vi "GetCtlRef_Base.vi"(8 "error in (no error)":errorcluster, 10 "Control Label":string, 11 "CtlLookup In":T1) -> (0 "error out":errorcluster, 2 "CtlRef Out":refnum<vi>, 3 "CtlLookup Out":T1)   [LabVIEW 2018, in "CtlReferences.lvlib" / "CtlReferences.lvclass"]
doc: "This is the base of the polymorphic VI \"GetControlRef\" \n\nThis is a General Helper VI.\n\nThis will search the incoming \"Ref Cluster\" for the Control Label string. If it finds it, it will output the reference If it does not, it will create an error -8000 with the control name"
uses:
  CtlReferences.lvclass
  TypeDefs/CtlLookup.ctl
  CtlReferences.lvclass/CtlReferences.ctl
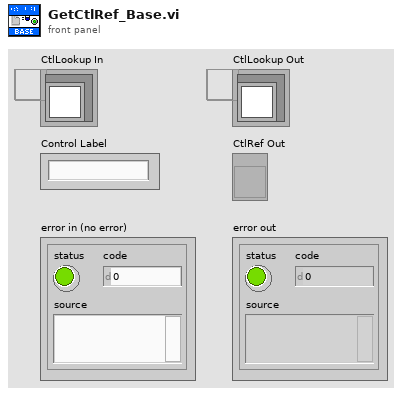
[diagram p1: front panel]
types:
  T1 = typedef "CtlReferences.lvlib/CtlReferences.lvclass/CtlLookup.ctl" = refnum<data-value>
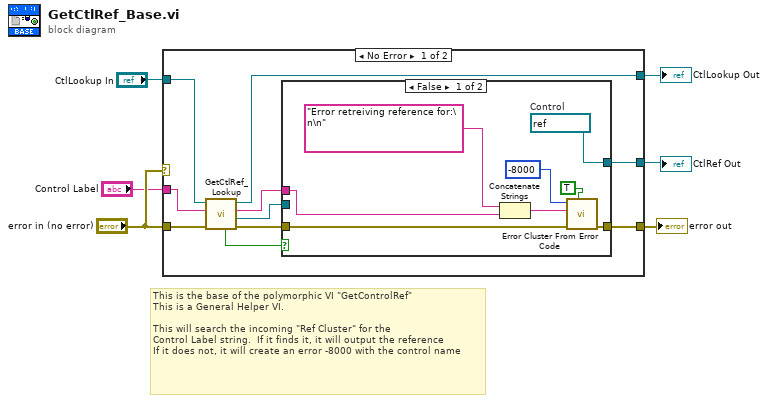
[diagram p0: block diagram]
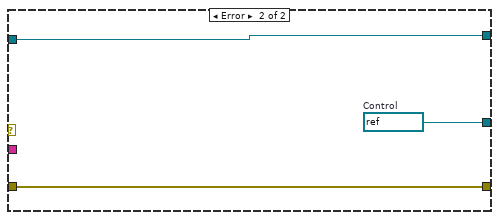
[diagram p3: hidden frame]
diagram:
  # "This is the base of the polymorphic VI \"GetControlRef\"\nThis is a General Helper VI.\n\nThis will search the incoming \"Ref Cluster\" for the \nControl Label string.  If it finds it, it will output the reference\nIf it does not, it will create an error -8000 with the control name"
  n1 = case shown="No Error" "error in (no error)" {
    tunnel: [w16 w29] -> w6
    tunnel: "error in (no error)" -> [w10 w29]
    tunnel: "CtlLookup In" -> [w15 w28]
    tunnel: [w13 w28] -> w3
    tunnel: [w12 w27] -> w2
    tunnel: "Control Label" -> [w14 _]
    frame No Error {
      n2 = call "GetCtlRef_Lookup.vi"("Error in"=w10, "CtlName In"=w14, "CtlLookup In"=w15) -> ("error out"=w11:errorcluster, "CtlRef"=w9:refnum<vi>, "CtlName Out"=w8:string, "CtlLookup Out"=w13:T1, "Control Label Found?"=w7:bool)  [unwired: 4 in]
      n3 = case shown="False" w7 {
        tunnel: w11 -> [w18 w26]
        tunnel: [w21 w26] -> w16
        tunnel: [w24 w25] -> w12
        tunnel: w8 -> [w22 _]
        tunnel: w9 -> [_ w25]
        frame False {
          w24 = refnum<vi> refnum  # Control
          n4 = Concatenate Strings("Error retreiving reference for:\n\n" ("source"), w22) -> (w20:string)
          n5 = call <vilib>:"Error Cluster From Error Code.vi"("show call chain? (False)"=TRUE ("Force Error? [F]"), "error in (no error)"=w18, "error message (\"\")"=w20, "error code (0)"=-8000 ("code")) -> ("error out"=w21:errorcluster)  [unwired: 5 in]
        }
        frame True {
        }
      }
    }
    frame Error {
      w27 = refnum<vi> refnum  # Control
    }
  }
  "error out" <- w6
  "CtlLookup Out" <- w3
  "CtlRef Out" <- w2
